vi "BRig_Host_dataRunState__entryDelete__delDataPlot_subunit1.vi"(9 "input_col_dataPlot":i32, 10 "input_row_dataPlot":i32, 11 "input_dataPlot":u16[][](array[numeric])) -> (3 "output_dataPlot":u16[][](array[numeric]))   [LabVIEW 2014]
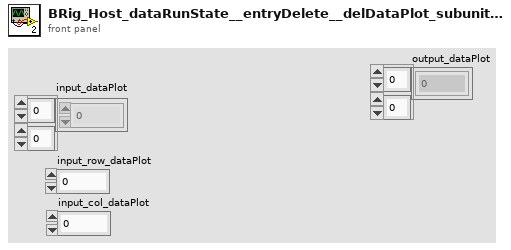
[diagram p1: front panel]
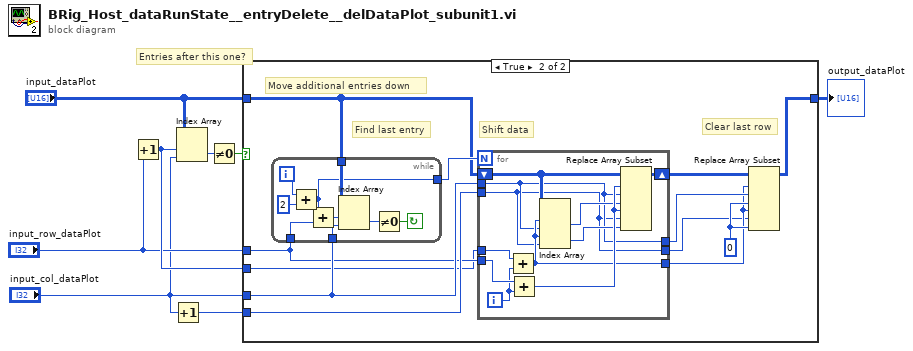
[diagram p0: block diagram]
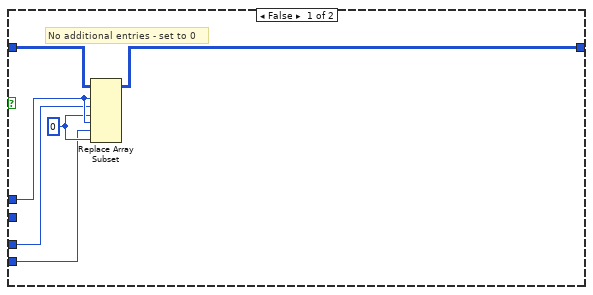
[diagram p2: hidden frame]
diagram:
  # "Entries after this one?"
  n1 = Increment(x="input_row_dataPlot") -> (x+1=w4:i32)
  n2 = Increment(x="input_col_dataPlot") -> (x+1=w5:i32)
  n3 = Index Array(array="input_dataPlot", index (row)=w4, index (col)="input_col_dataPlot") -> (element=w8:u16)
  n4 = Not Equal To 0?(x=w8) -> (x != 0?=w7:bool)
  n5 = case shown="True" w7 {
    tunnel: "input_dataPlot" -> [w14 w25]
    tunnel: "input_row_dataPlot" -> [w13 w22]
    tunnel: "input_col_dataPlot" -> [w12 w23]
    tunnel: [w10 w18] -> w3
    tunnel: w5 -> [w9 w24]
    tunnel: w4 -> [_ w21]
    frame False {
      w11 = u16 0 ("new element/subarray")
      # "No additional entries - set to 0"
      n6 = Replace Array Subset(array=w14, new element #1=w11, index (row) #1=w13, index (col) #1=w12, new element #2=w11, index (row) #2=w13, index (col) #2=w9) -> (w10:u16[][])
    }
    frame True {
      w20 = u16 0 ("new element/subarray")
      # "Clear last row"
      # "Shift data"
      # "Find last entry"
      # "Move additional entries down"
      n7 = while {
        tunnel: w25 -> [w46]
        tunnel: w23 -> [w43]
        tunnel: w22 -> [w40]
        tunnel: [w39] -> w26
        i -> [w42]
        stop <- w45 continue-if-true
        n8 = Add(x=w42, y=2) -> (x+y=w39:i32)
        n9 = Add(x=w39, y=w40) -> (x+y=w38:i32)
        n10 = Index Array(array=w46, index (row)=w38, index (col)=w43) -> (element=w44:u16)
        n11 = Not Equal To 0?(x=w44) -> (x != 0?=w45:bool)
      }
      n12 = for {
        N: w26 -> [_]
        shift-right: [w37] -> w19
        shift-left: w25 -> [w36]
        tunnel: w22 -> [w35]
        tunnel: w21 -> [w33]
        tunnel: w23 -> [w28]
        tunnel: w24 -> [w27]
        tunnel: [w29] -> w16
        tunnel: [w28] -> w17
        tunnel: [w27] -> w15
        i -> [w34]
        n13 = Add(x=w33, y=w34) -> (x+y=w29:i32)
        n14 = Add(x=w35, y=w34) -> (x+y=w32:i32)
        n15 = Index Array(array=w36, index (row) #1=w29, index (col) #1=w28, index (row) #2=w29, index (col) #2=w27) -> (element #1=w31:u16, element #2=w30:u16)
        n16 = Replace Array Subset(array=w36, new element #1=w31, index (row) #1=w32, index (col) #1=w28, new element #2=w30, index (row) #2=w32, index (col) #2=w27) -> (w37:u16[][])
      }
      n17 = Replace Array Subset(array=w19, new element #1=w20, index (row) #1=w16, index (col) #1=w17, new element #2=w20, index (row) #2=w16, index (col) #2=w15) -> (w18:u16[][])
    }
  }
  "output_dataPlot" <- w3
